vi "NIDCPower_channel_ganging - configure voltage level.vi"(8 "error in (no error)":errorcluster, 9 "voltage level":dbl format="%_6p", 11 "Ganged Session In":T1) -> (0 "error out":errorcluster, 3 "Ganged Session Out":T1)   [LabVIEW 2024]
uses:
  ctl/NIDCPower_channel_ganging - ctl - ganged session.ctl
  ctl/NIDCPower_channel_ganging - ctl - ganged config.ctl
  ctl/NIDCPower_channel_ganging - ctl - channel mode.ctl
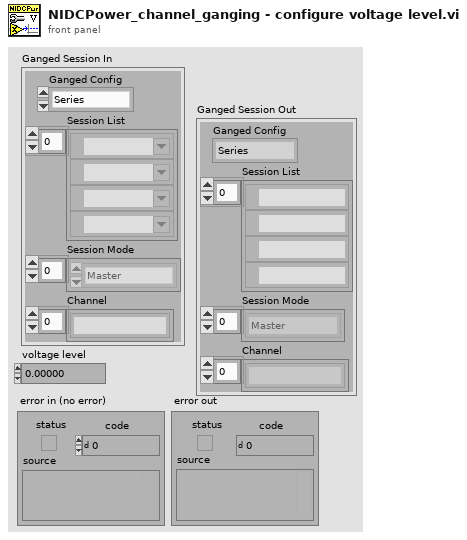
[diagram p1: front panel]
types:
  T1 = typedef "NIDCPower_channel_ganging - ctl - ganged session.ctl" = cluster{"Ganged Config":T2, "Session List":refnum<k15>[], "Session Mode":T3[], "Channel":string[]}
  T2 = typedef "NIDCPower_channel_ganging - ctl - ganged config.ctl" = enum32{"Series", "Parallel", "Manual"}
  T3 = typedef "NIDCPower_channel_ganging - ctl - channel mode.ctl" = enum32{"Master", "Slave", "Slave - Inverted"}
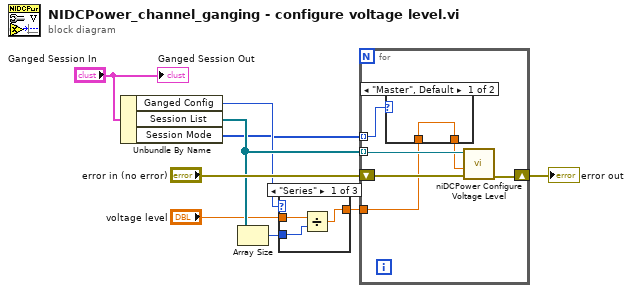
[diagram p0: block diagram]
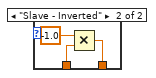
[diagram p4: hidden frame]
diagram:
  n1 = Unbundle By Name("Ganged Session In") -> ("Ganged Config"=w5:T2, "Session List"=w6:refnum<k15>[], "Session Mode"=w1:T3[])
  n2 = Array Size(array=w6) -> (size(s)=w4:i32)
  n3 = case shown="\"Series\"" w5 {
    tunnel: w4 -> [w11 _ _]
    tunnel: "voltage level" -> [w12 w13 w14]
    tunnel: [w10 w13 w14] -> w2
    frame "Series" {
      n4 = Divide(x=w12, y=w11) -> (x/y=w10:dbl)
    }
    frame "Parallel" {
    }
    frame "Manual" {
    }
  }
  n5 = for {
    shift-right: [w15] -> w8
    shift-left: "error in (no error)" -> [w20]
    tunnel: w6 -> [w19] mode=indexing
    tunnel: w2 -> [w16]
    tunnel: w1 -> [w18] mode=indexing
    n6 = case shown="\"Master\", Default" w18 {
      tunnel: w16 -> [w21 w24]
      tunnel: [w21 w23] -> w17
      frame "Master", Default {
      }
      frame "Slave - Inverted" {
        n7 = Multiply(x=-1.0, y=w24) -> (x*y=w23:dbl)
      }
    }
    n8 = call <instrlib>:"niDCPower Configure Voltage Level.vi"("error in (no error)"=w20, "voltage level"=w17, "instrument handle"=w19) -> ("error out"=w15:errorcluster)  [unwired: 7 in, 1 out]
  }
  "error out" <- w8
  "Ganged Session Out" <- "Ganged Session In"
